vi "Configure Constant Power.vi"(6 "Desired Power (0.00 W)":dbl format="%_3g", 7 "Overvoltage Protection Value (0.00 V)":dbl format="%_3g", 8 "error in (no error)":errorcluster, 9 "Maximum Current (0.00 A)":dbl format="%_3g", 10 "Maximum Voltage (0.00 V)":dbl format="%_3g", 11 "VISA resource name":refnum<visa-resource-name>) -> (0 "error out":errorcluster, 3 "VISA resource name out":refnum<visa-resource-name>)   [LabVIEW 2020, in "Sorensen SG Series.lvlib"]
doc: "Places the instrument into a constant power state, where voltage and current are varied to maintain this value if necessary."
uses:
  <instrlib>/Sorensen SG Series/Sorensen SG Series.lvlib
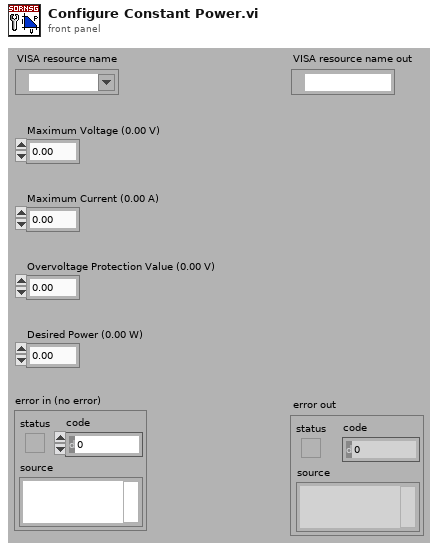
[diagram p1: front panel]
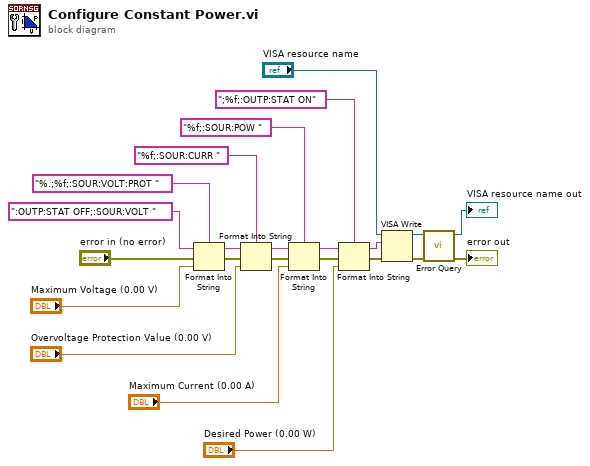
[diagram p0: block diagram]
diagram:
  n1 = Format Into String(format string="%.;%f;:SOUR:VOLT:PROT ", initial string=":OUTP:STAT OFF;:SOUR:VOLT ", error in="error in (no error)", "Maximum Voltage (0.00 V)") -> (resulting string=w18:string, error out=w19:errorcluster)
  n2 = Format Into String(format string="%f;:SOUR:CURR ", initial string=w18, error in=w19, "Overvoltage Protection Value (0.00 V)") -> (resulting string=w14:string, error out=w15:errorcluster)
  n3 = Format Into String(format string="%f;:SOUR:POW ", initial string=w14, error in=w15, "Maximum Current (0.00 A)") -> (resulting string=w10:string, error out=w11:errorcluster)
  n4 = Format Into String(format string=";%f;:OUTP:STAT ON", initial string=w10, error in=w11, "Desired Power (0.00 W)") -> (resulting string=w8:string, error out=w6:errorcluster)
  n5 = VISA Write(VISA resource name="VISA resource name", write buffer=w8, error in (no error)=w6) -> (VISA resource name out=w4:refnum<visa-resource-name>, error out=w5:errorcluster)  [unwired: 1 out]
  n6 = call <instrlib>:"Error Query.vi"("error in (no error)"=w5, "VISA resource name"=w4) -> ("error out"=→"error out":errorcluster, "VISA resource name out"=→"VISA resource name out":refnum<visa-resource-name>)  [unwired: 6 in, 2 out]
